vi "HexToWord.vi"(11 "Registers":u16[](array[numeric]) format="%xH") -> (3 "数组":u16[](array[numeric]))   [LabVIEW 2016, in "超标留样集成.lvlib" / "ESTD1200.lvlib"]
uses:
  ESTD1200.lvlib
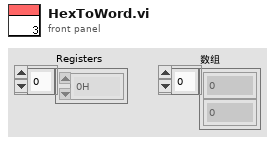
[diagram p1: front panel]
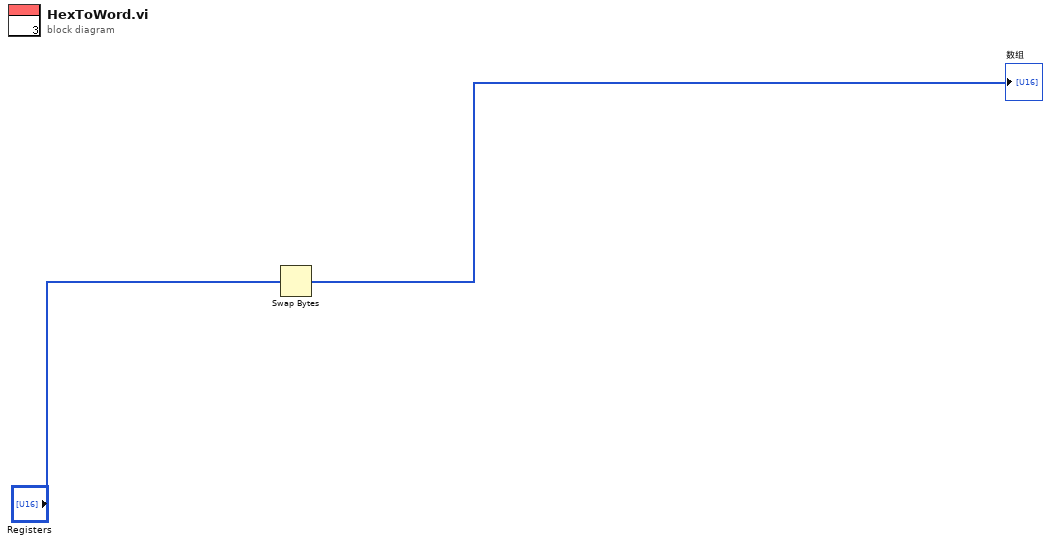
[diagram p0: block diagram]
diagram:
  n1 = Swap Bytes(anything="Registers") -> (byte swapped=→"数组":u16[])
